vi "getLHeLevel.vi"(8 "error in (no error)":errorcluster, 11 "Instrument.Oxford1820 in":refnum<class "Instrument.Oxford1820.lvclass">) -> (0 "error out":errorcluster, 2 "LHe Level (%)":dbl, 3 "Instrument.Oxford1820 out":refnum<class "Instrument.Oxford1820.lvclass">)   [LabVIEW 2019, in "Instrument.Oxford1820.lvclass"]
uses:
  Instrument.Oxford1820.lvclass
  Typedefs/Instrument.Oxford1820.publicCommands-enum.ctl
  Typedefs/getLHeLevel--Cluster.ctl
  399ad0ad-0d21-49b5-a294-8196154d3987.vi
  399ad0ad-0d21-49b5-a294-8196154d3987.vi/949acce6-d728-4655-9172-581a69a31cf6.vi
  399ad0ad-0d21-49b5-a294-8196154d3987.vi/2bea5523-4ada-4b31-8337-7c648f53c0ab.vi
  <vilib>/Utility/Data Type/Get Type Information.vi
  <vilib>/JDP Science/JSONtext/JSON text to Variant.vi
  <vilib>/JDP Science/JSONtext/LVClass Serializer/JSONtext LVClass Serializer.lvclass
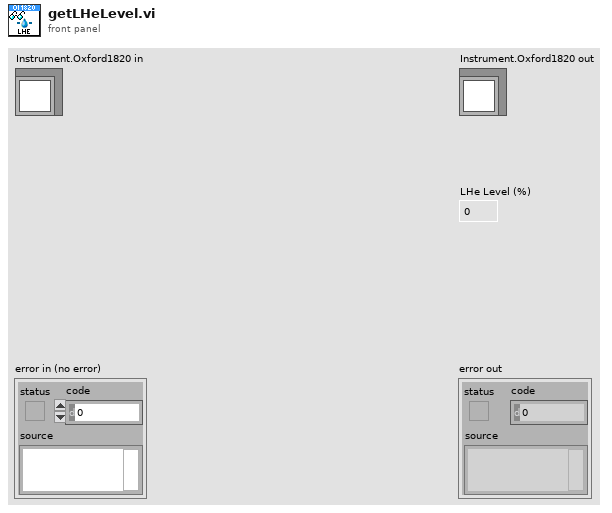
[diagram p1: front panel]
types:
  T1 = typedef "Instrument.Oxford1820.lvclass/getLHeLevel--Cluster.ctl" = cluster{"LHeLevel":dbl}
  T2 = typedef "Instrument.Oxford1820.lvclass/Instrument.Oxford1820.publicCommands-enum.ctl" = enum16{"setMagnet", "getMagnet", "getMagnetTarget", "getLHeLevel", "getLN2level"}
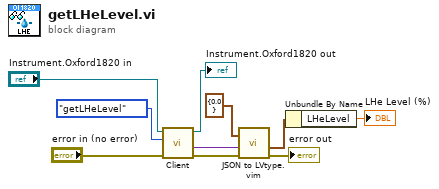
[diagram p0: block diagram]
diagram:
  n1 = call-dynamic "Client.vi"("error in (no error)"="error in (no error)", "Command in"=Instrument.Oxford1820.publicCommands-enum."getLHeLevel" ("publicCommands"), "Instrument in"="Instrument.Oxford1820 in") -> ("error out"=w4:errorcluster, "Data out"=w5:variant, "Instrument out"=→"Instrument.Oxford1820 out":refnum<class "Instrument.Oxford1820.lvclass">)  [unwired: 5 in, 1 out]
  n2 = call "JSON to LVtype.vim"("type"=T1 {"LHeLevel"=0.0} ("getHeLevel"), "error in (no error)"=w4, "JSON Data in"=w5) -> ("error out"=→"error out":errorcluster, "Data out"=w3:T1)  [unwired: 7 in]
  n3 = Unbundle By Name(w3) -> ("LHeLevel"=→"LHe Level (%)":dbl)
